vi "Revision Query.vi"(8 "error in (no error)":errorcluster, 11 "IVI_DCPwr in":refnum<class "IVI_DCPwr.lvclass">) -> (0 "error out":errorcluster, 1 "Firmware Revision":string, 2 "Driver Revision":string, 3 "IVI_DCPwr out":refnum<class "IVI_DCPwr.lvclass">)   [LabVIEW 2013, in "IVI_DCPwr.lvlib" / "IVI_DCPwr.lvclass"]
uses:
  IVI_DCPwr.lvclass
  IVI_DCPwr.lvclass/IVI_DCPwr.ctl
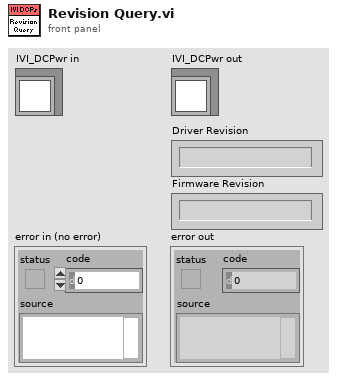
[diagram p1: front panel]
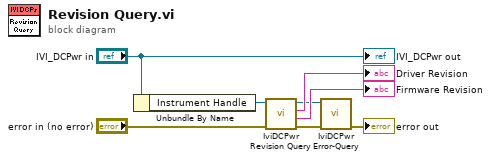
[diagram p0: block diagram]
diagram:
  n1 = Unbundle By Name("IVI_DCPwr in") -> ("Instrument Handle"=w7:refnum<k15>)
  n2 = call <vilib>:"IviDCPwr Revision Query.vi"("error in (no error)"="error in (no error)", "instrument handle"=w7) -> ("error out"=w2:errorcluster, "firmware revision"=→"Firmware Revision":string, "instrument driver revision"=→"Driver Revision":string, "instrument handle out"=w3:refnum<k15>)  [unwired: 6 in]
  n3 = call <vilib>:"IviDCPwr Error-Query.vi"("error in (no error)"=w2, "instrument handle"=w3) -> ("error out"=→"error out":errorcluster)  [unwired: 6 in, 3 out]
  "IVI_DCPwr out" <- "IVI_DCPwr in"
